vi "KB-C Chart.vi"(9 "P Chart Select":string(combo)="ITEM31(Offset)O-I", 10 "ALL Tolerance Param":string[][](table)=[["Null", "Null", "Null", "Null", "Null", "Null", "Null", "Null", "Null"], ["Null", "Null", "Null", "Null", "Null", "Null", "Null", "Null", "Null"], ["Null", "Null", "Null", "Null", "Null", "Null", "Null", "Null", "Null"], ["Null", "Null", "Null", "Null", "Null", "Null", "Null", "Null", "Null"], ["Null", "Null", "Null", "Null", "Null", "Null", "Null", "Null", "Null"], ["Null", "Null", "Null", "Null", "Null", "Null", "Null", "Null", "Null"], ["Null", "Null", "Null", "Null", "Null", "Null", "Null", "Null", "Null"], ["Null", "Null", "Null", "Null", "Null", "Null", "Null", "Null", "Null"], ["Null", "Null", "Null", "Null", "Null", "Null", "Null", "Null", "Null"], ["Null", "Null", "Null", "Null", "Null", "Null", "Null", "Null", "Null"], ["Null", "Null", "Null", "Null", "Null", "Null", "Null", "Null", "Null"], ["Null", "Null", "Null", "Null", "Null", "Null", "Null", "Null", "Null"], ["Null", "Null", "Null", "Null", "Null", "Null", "Null", "Null", "Null"], ["Null", "Null", "Null", "Null", "Null", "Null", "Null", "Null", "Null"], ["Null", "Null", "Null", "Null", "Null", "Null", "Null", "Null", "Null"], ["Null", "Null", "Null", "Null", "Null", "Null", "Null", "Null", "Null"], ["Null", "Null", "Null", "Null", "Null", "Null", "Null", "Null", "Null"], ["Null", "Null", "Null", "Null", "Null", "Null", "Null", "Null", "Null"], ["Null", "Null", "Null", "Null", "Null", "Null", "Null", "Null", "Null"], ["Null", "Null", "Null", "Null", "Null", "Null", "Null", "Null", "Null"], ["Null", "Null", "Null", "Null", "Null", "Null", "Null", "Null", "Null"], ["Null", "Null", "Null", "Null", "Null", "Null", "Null", "Null", "Null"], ["Null", "Null", "Null", "Null", "Null", "Null", "Null", "Null", "Null"], ["Null", "Null", "Null", "Null", "Null", "Null", "Null", "Null", "Null"], ["Null", "Null", "Null", "Null", "Null", "Null", "Null", "Null", "Null"], ["Null", "Null", "Null", "Null", "Null", "Null", "Null", "Null", "Null"], ["Null", "Null", "Null", "Null", "Null", "Null", "Null", "Null", "Null"], ["Null", "Null", "Null", "Null", "Null", "Null", "Null", "Null", "Null"], ["Null", "Null", "Null", "Null", "Null", "Null", "Null", "Null", "Null"], ["Null", "Null", "Null", "Null", "Null", "Null", "Null", "Null", "Null"], ["Null", "Null", "Null", "Null", "Null", "Null", "Null", "Null", "Null"], ["Null", "Null", "Null", "Null", "Null", "Null", "Null", "Null", "Null"], ["Null", "Null", "Null", "Null", "Null", "Null", "Null", "Null", "Null"]], 11 "Data":string[][](table)=[["Barcode", "StartTime", "Result", "ProductColor", "ITEM1 Result", "ITEM1(Offset)O-I", "ITEM1(Offset)I", "ITEM1(Offset)O", "ITEM1同心度", "ITEM1颜色", "ITEM1是否漏装", "ITEM2 Result", "ITEM2(Offset)O-I", "ITEM2(Offset)I", "ITEM2(Offset)O", "ITEM2同心度", "ITEM2颜色", "ITEM2是否漏装", "ITEM3 Result", "ITEM3(Offset)O-I", "ITEM3(Offset)I", "ITEM3(Offset)O", "ITEM3同心度", "ITEM3颜色", "ITEM3是否漏装", "ITEM4 Result", "ITEM4(Offset)O-I", "ITEM4(Offset)I", "ITEM4(Offset)O", "ITEM4同心度", "ITEM4颜色", "ITEM4是否漏装", "ITEM5 Result", "ITEM5(Offset)O-I", "ITEM5(Offset)I", "ITEM5(Offset)O", "ITEM5同心度", "ITEM5颜色", "ITEM5是否漏装", "ITEM6 Result", "ITEM6(Offset)O-I", "ITEM6(Offset)I", "ITEM6(Offset)O", "ITEM6同心度", "ITEM6颜色", "ITEM6是否漏装", "ITEM7 Result", "ITEM7(Offset)O-I", "ITEM7(Offset)I", "ITEM7(Offset)O", "ITEM7同心度", "ITEM7颜色", "ITEM7是否漏装", "ITEM8 Result", "ITEM8(Offset)O-I", "ITEM8(Offset)I", "ITEM8(Offset)O", "ITEM8同心度", "ITEM8颜色", "ITEM8是否漏装", "ITEM9 Result", "ITEM9(Offset)O-I", "ITEM9(Offset)I", "ITEM9(Offset)O", "ITEM9同心度", "ITEM9颜色", "ITEM9是否漏装", "ITEM10 Result", "ITEM10(Offset)O-I", "ITEM10(Offset)I", "ITEM10(Offset)O", "ITEM10同心度", "ITEM10颜色", "ITEM10是否漏装", "ITEM11 Result", "ITEM11(Offset)O-I", "ITEM11(Offset)I", "ITEM11(Offset)O", "ITEM11同心度", "ITEM11颜色", "ITEM11是否漏装", "ITEM12 Result", "ITEM12(Offset)O-I", "ITEM12(Offset)I", "ITEM12(Offset)O", "ITEM12同心度", "ITEM12颜色", "ITEM12是否漏装", "ITEM13 Result", "ITEM13(Offset)O-I", "ITEM13(Offset)I", "ITEM13(Offset)O", "ITEM13同心度", "ITEM13颜色", "ITEM13是否漏装", "ITEM14 Result", "ITEM14(Offset)O-I", "ITEM14(Offset)I", "ITEM14(Offset)O", "ITEM14同心度", "ITEM14颜色", "ITEM14是否漏装", "ITEM15 Result", "ITEM15(Offset)O-I", "ITEM15(Offset)I", "ITEM15(Offset)O", "ITEM15同心度", "ITEM15颜色", "ITEM15是否漏装", "ITEM16 Result", "ITEM16(Offset)O-I", "ITEM16(Offset)I", "ITEM16(Offset)O", "ITEM16同心度", "ITEM16颜色", "ITEM16是否漏装", "ITEM17 Result", "ITEM17(Offset)O-I", "ITEM17(Offset)I", "ITEM17(Offset)O", "ITEM17同心度", "ITEM17颜色", "ITEM17是否漏装", "ITEM18 Result", "ITEM18(Offset)O-I", "ITEM18(Offset)I", "ITEM18(Offset)O", "ITEM18同心度", "ITEM18颜色", "ITEM18是否漏装", "ITEM19 Result", "ITEM19(Offset)O-I", "ITEM19(Offset)I", "ITEM19(Offset)O", "ITEM19同心度", "ITEM19颜色", "ITEM19是否漏装", "ITEM20 Result", "ITEM20(Offset)O-I", "ITEM20(Offset)I", "ITEM20(Offset)O", "ITEM20同心度", "ITEM20颜色", "ITEM20是否漏装", "ITEM21 Result", "ITEM21(Offset)O-I", "ITEM21(Offset)I", "ITEM21(Offset)O", "ITEM21同心度", "ITEM21颜色", "ITEM21是否漏装", "ITEM22 Result", "ITEM22(Offset)O-I", "ITEM22(Offset)I", "ITEM22(Offset)O", "ITEM22同心度", "ITEM22颜色", "ITEM22是否漏装", "ITEM23 Result", "ITEM23(Offset)O-I", "ITEM23(Offset)I", "ITEM23(Offset)O", "ITEM23同心度", "ITEM23颜色", "ITEM23是否漏装", "ITEM24 Result", "ITEM24(Offset)O-I", "ITEM24(Offset)I", "ITEM24(Offset)O", "ITEM24同心度", "ITEM24颜色", "ITEM24是否漏装", "ITEM25 Result", "ITEM25(Offset)O-I", "ITEM25(Offset)I", "ITEM25(Offset)O", "ITEM25同心度", "ITEM25颜色", "ITEM25是否漏装", "ITEM26 Result", "ITEM26(Offset)O-I", "ITEM26(Offset)I", "ITEM26(Offset)O", "ITEM26同心度", "ITEM26颜色", "ITEM26是否漏装", "ITEM27 Result", "ITEM27(Offset)O-I", "ITEM27(Offset)I", "ITEM27(Offset)O", "ITEM27同心度", "ITEM27颜色", "ITEM27是否漏装", "ITEM28 Result", "ITEM28(Offset)O-I", "ITEM28(Offset)I", "ITEM28(Offset)O", "ITEM28同心度", "ITEM28颜色", "ITEM28是否漏装", "ITEM29 Result", "ITEM29(Offset)O-I", "ITEM29(Offset)I", "ITEM29(Offset)O", "ITEM29同心度", "ITEM29颜色", "ITEM29是否漏装", "ITEM30 Result", "ITEM30(Offset)O-I", "ITEM30(Offset)I", "ITEM30(Offset)O", "ITEM30同心度", "ITEM30颜色", "ITEM30是否漏装", "ITEM31 Result", "ITEM31(Offset)O-I", "ITEM31(Offset)I", "ITEM31(Offset)O", "ITEM31同心度", "ITEM31颜色", "ITEM31是否漏装"], ["3434", "2016-09-24 08:24:53 +0800", "NG", "白色", "OK", "0.040", "0.013", "Null", "0.061", "金色", "无漏装", "OK", "0.059", "0.016", "Null", "0.031", "金色", "无漏装", "OK", "0.042", "0.002", "Null", "0.031", "金色", "无漏装", "OK", "0.056", "0.016", "Null", "0.019", "金色", "无漏装", "OK", "0.037", "0.017", "Null", "0.024", "金色", "无漏装", "OK", "0.059", "0.019", "Null", "0.028", "金色", "无漏装", "OK", "Null", "Null", "Null", "0", "银色", "无漏装", "OK", "Null", "Null", "Null", "0", "银色", "无漏装", "OK", "Null", "Null", "Null", "0", "银色", "无漏装", "OK", "Null", "Null", "Null", "0", "银色", "无漏装", "OK", "0.106", "0.000", "Null", "0.039", "金色", "无漏装", "OK", "0.099", "0.012", "Null", "0.060", "金色", "无漏装", "OK", "0.071", "0.006", "Null", "0.064", "金色", "无漏装", "OK", "0.086", "0.020", "Null", "0.027", "金色", "无漏装", "OK", "0.098", "0.005", "Null", "0.047", "金色", "无漏装", "高度差NG", "-0.027", "0.000", "Null", "0.067", "金色", "无漏装", "OK", "0.081", "0.002", "Null", "0.050", "金色", "无漏装", "OK", "0.102", "0.016", "Null", "0.018", "金色", "无漏装", "OK", "0.154", "0.013", "Null", "0.048", "金色", "无漏装", "OK", "0.040", "0.004", "Null", "0.036", "金色", "无漏装", "OK", "0.065", "0.014", "Null", "0.030", "金色", "无漏装", "OK", "0.205", "0.004", "1.260", "0.015", "金色", "无漏装", "高度差NG", "0.302", "0.006", "0.921", "0.023", "金色", "无漏装", "OK", "0.150", "0.009", "1.375", "0.018", "金色", "无漏装", "高度差NG", "0.267", "0.006", "0.913", "0.034", "金色", "无漏装", "OK", "0.147", "0.016", "0.936", "0.048", "金色", "无漏装", "OK", "0.198", "0.012", "1.345", "0.003", "金色", "无漏装", "高度差NG", "0.350", "0.017", "1.198", "0.037", "金色", "无漏装", "高度差NG", "0.387", "0.011", "0.924", "0.015", "金色", "无漏装", "OK", "0.125", "0.007", "0.962", "0.023", "金色", "无漏装", "高度差NG", "0.289", "0.014", "1.281", "0.021", "金色", "无漏装"]]) -> (3 "结果直方图":dbl[][](graph)=[[0.0, 0.136, 0.145, 0.129, 0.138, 0.133, 0.115, 0.126, 0.122, 0.132, 0.133, 0.133, 0.113, 0.108, 0.111, 0.181, 0.185, 0.182, 0.224, 0.217, 0.221, 0.187, 0.192, 0.188, 0.187, 0.188, 0.19, 0.137, 0.136, 0.134, 0.202, 0.202, 0.206, 0.037, 0.038, 0.036], [0.25, 0.25, 0.25, 0.25, 0.25, 0.25, 0.25, 0.25, 0.25, 0.25, 0.25, 0.25, 0.25, 0.25, 0.25, 0.25, 0.25, 0.25, 0.25, 0.25, 0.25, 0.25, 0.25, 0.25, 0.25, 0.25, 0.25, 0.25, 0.25, 0.25, 0.25, 0.25, 0.25, 0.25, 0.25, 0.25], [0.0, 0.0, 0.0, 0.0, 0.0, 0.0, 0.0, 0.0, 0.0, 0.0, 0.0, 0.0, 0.0, 0.0, 0.0, 0.0, 0.0, 0.0, 0.0, 0.0, 0.0, 0.0, 0.0, 0.0, 0.0, 0.0, 0.0, 0.0, 0.0, 0.0, 0.0, 0.0, 0.0, 0.0, 0.0, 0.0], [0.125, 0.125, 0.125, 0.125, 0.125, 0.125, 0.125, 0.125, 0.125, 0.125, 0.125, 0.125, 0.125, 0.125, 0.125, 0.125, 0.125, 0.125, 0.125, 0.125, 0.125, 0.125, 0.125, 0.125, 0.125, 0.125, 0.125, 0.125, 0.125, 0.125, 0.125, 0.125, 0.125, 0.125, 0.125, 0.125]])   [LabVIEW 2015]
panel:
  out "添加的数组 2":i32[](array[numeric])
  out "数字":dbl[](array[numeric])
  out "添加的数组":i32[](array[numeric])
  out "大小 2":i32
  out "大小":i32
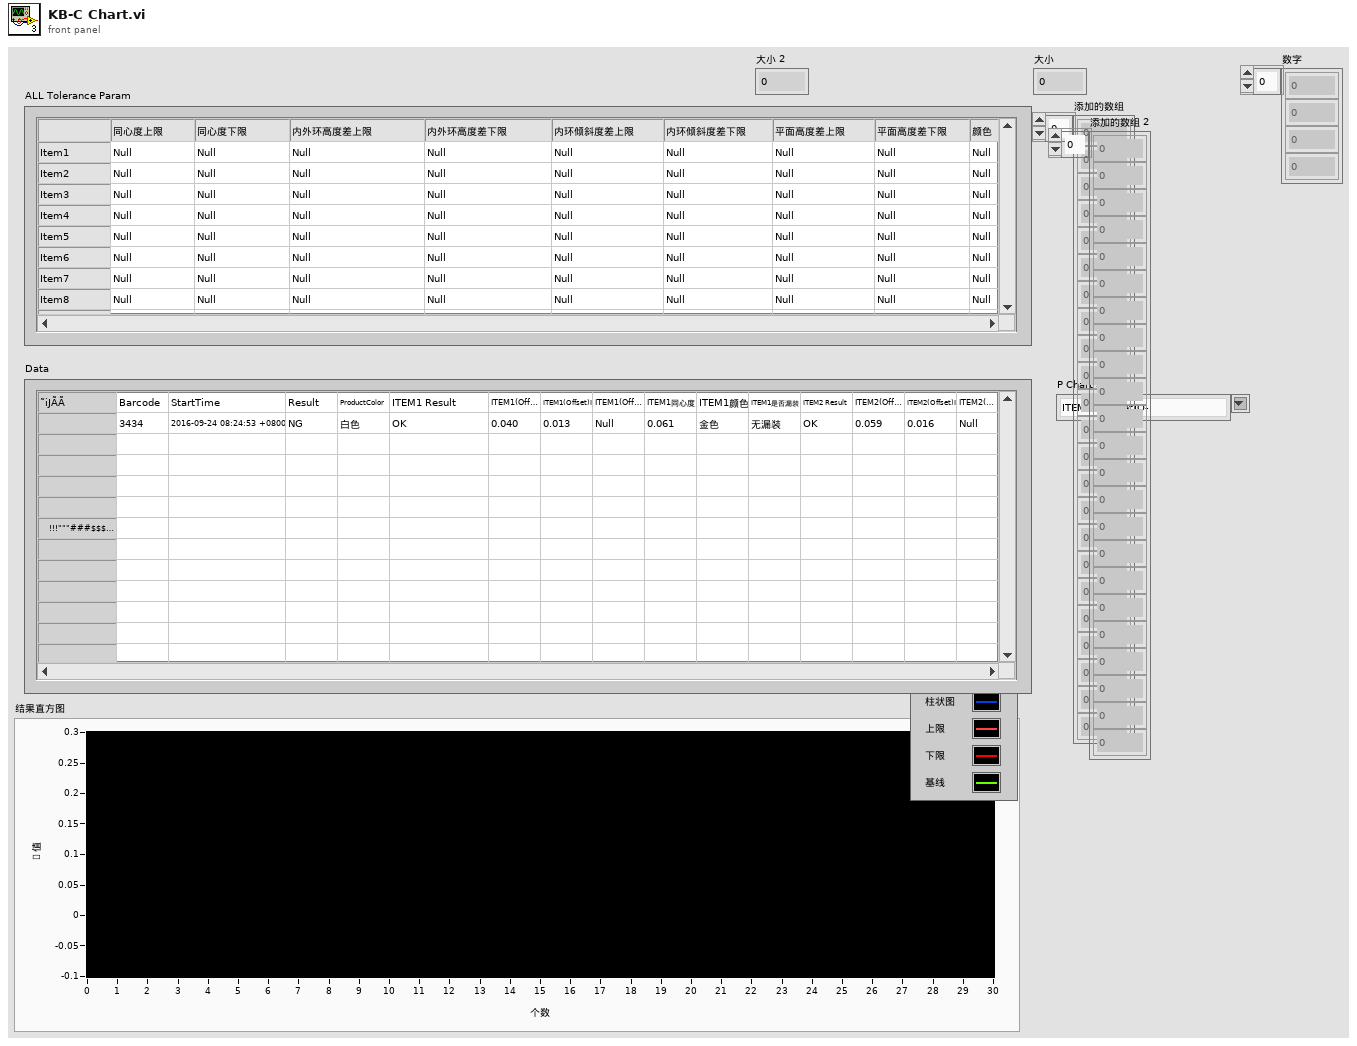
[diagram p1: front panel]
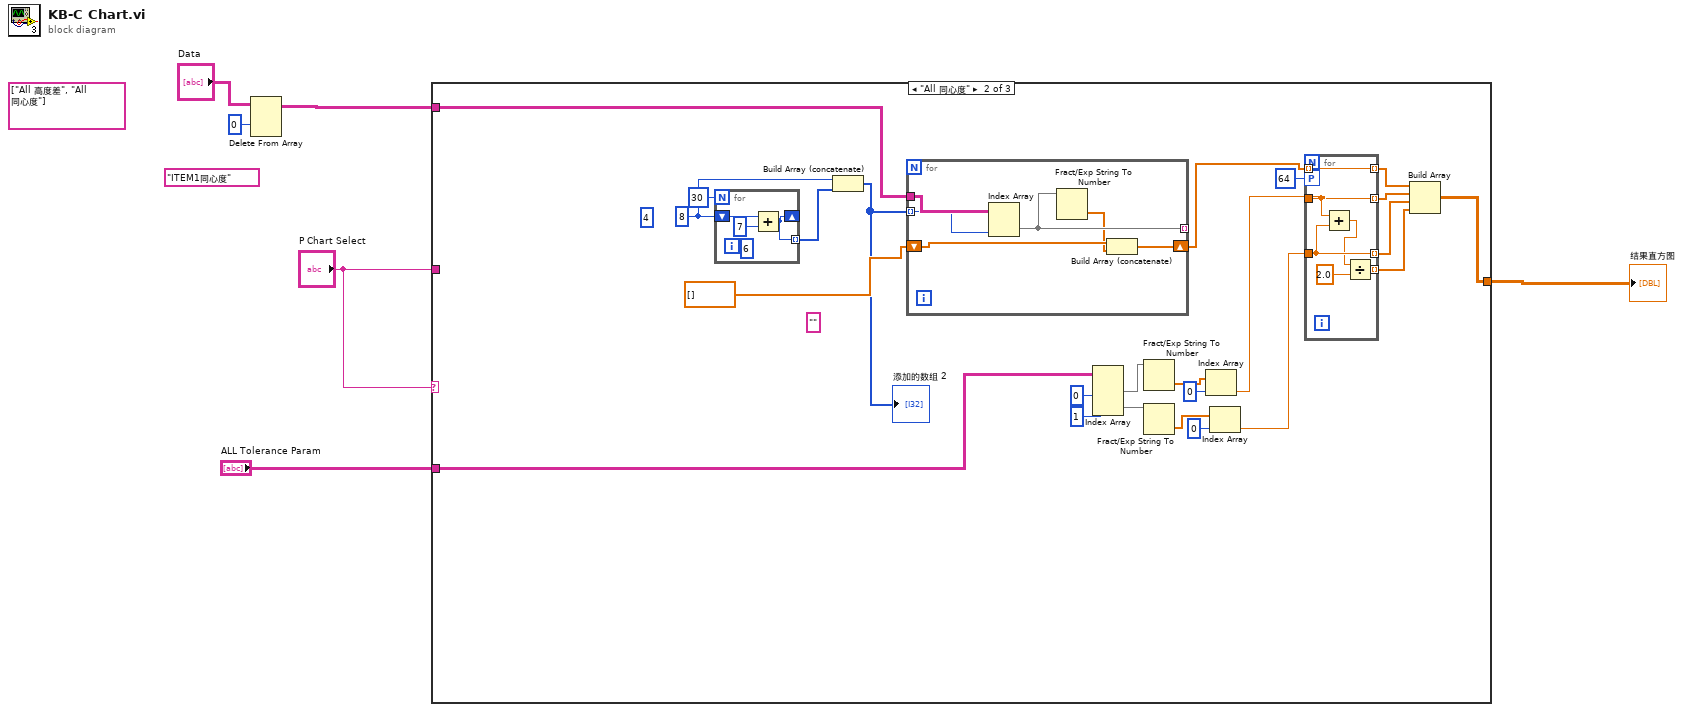
[diagram p0: block diagram]
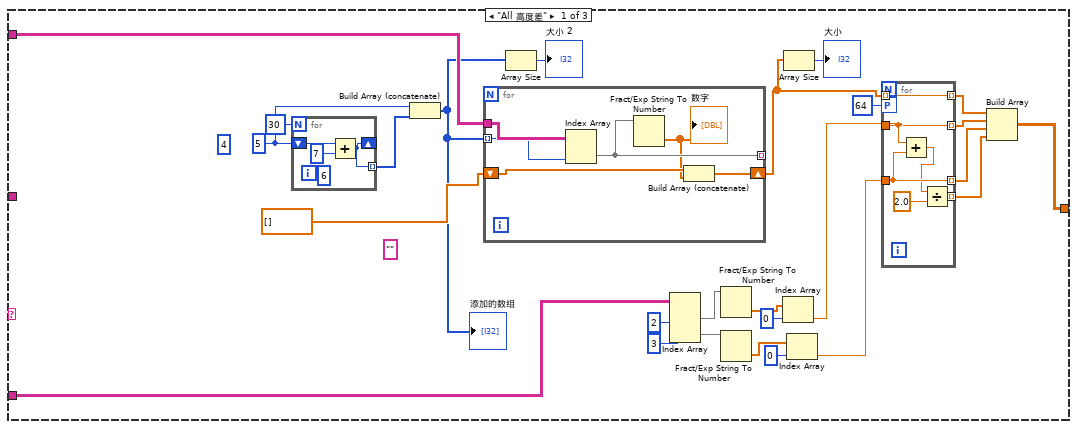
[diagram p2: hidden frame]
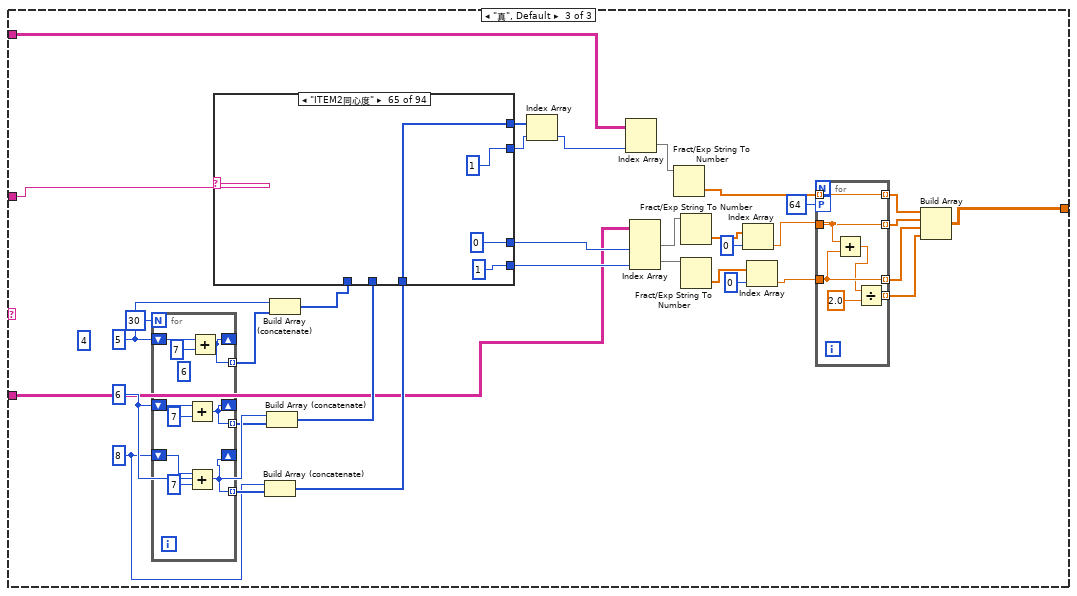
[diagram p3: hidden frame]
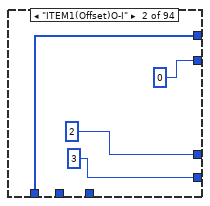
[diagram p5: hidden frame]
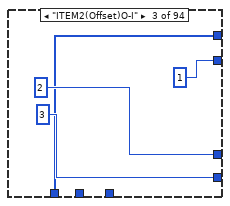
[diagram p6: hidden frame]
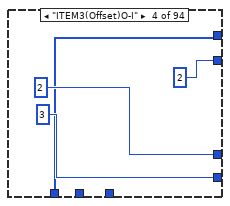
[diagram p7: hidden frame]
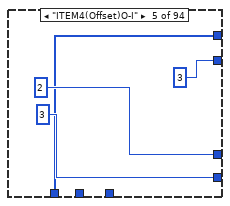
[diagram p8: hidden frame]
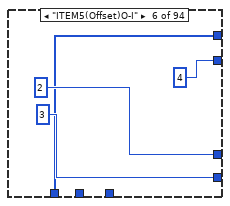
[diagram p9: hidden frame]
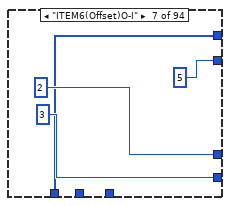
[diagram p10: hidden frame]
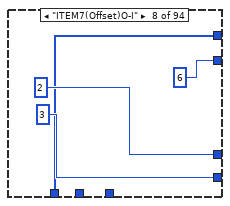
[diagram p11: hidden frame]
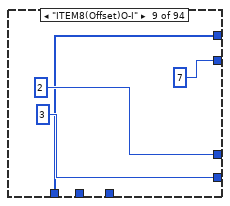
[diagram p12: hidden frame]
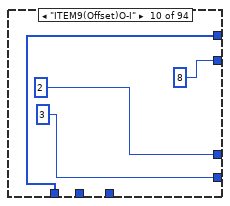
[diagram p13: hidden frame]
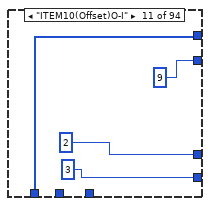
[diagram p14: hidden frame]
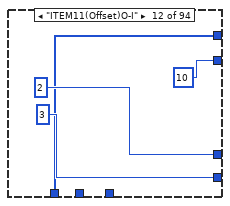
[diagram p15: hidden frame]
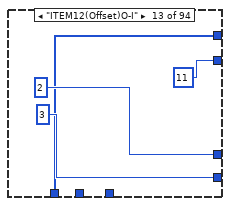
[diagram p16: hidden frame]
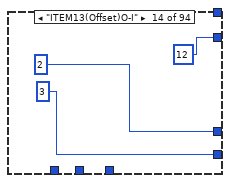
[diagram p17: hidden frame]
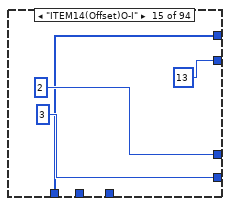
[diagram p18: hidden frame]
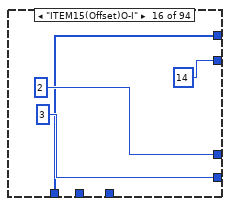
[diagram p19: hidden frame]
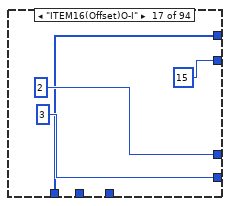
[diagram p20: hidden frame]
diagram:
  (unwired) string[] ["All 高度差", "All 同心度"] ("元素")
  (unwired) "ITEM1同心度" ("P Chart Select 2")
  n1 = Delete From Array(array="Data", index (row)=0 ("索引 (行)")) -> (array with subset deleted=w1:string[][])  [unwired: 2 in, 1 out]
  n2 = case shown="\"All 同心度\"" "P Chart Select" {
    tunnel: [w11 w50 w107] -> w6
    tunnel: w1 -> [w29 w68 w95]
    tunnel: "P Chart Select" -> [_ _ w94]
    tunnel: "ALL Tolerance Param" -> [w22 w61 w87]
    frame "All 高度差" {
      (unwired) ""
      (unwired) 4
      w30 = 5
      n3 = for {
        N: 30 -> [_]
        shift-right: [w45] -> _
        shift-left: w30 -> [w47]
        tunnel: [w45] -> w31 mode=indexing
        (unwired) 6 ("y")
        n4 = Add(x=w47, y=7) -> (x+y=w45:i32)
      }
      n5 = Build Array (concatenate)(w30, w31) -> (w7:i32[])
      "添加的数组" <- w7
      n6 = for {
        tunnel: w7 -> [w43] mode=indexing
        tunnel: w29 -> [w44]
        tunnel: [w41] -> _ mode=indexing
        shift-right: [w39] -> w10
        shift-left: dbl[] [] -> [w42]
        n7 = Index Array(array=w44, index (col)=w43) -> (element=w41:string[])  [unwired: 1 in]
        n8 = Fract/Exp String To Number ("分数/指数字符串至数值转换")(string=w41) -> (number=w40:dbl[])  [unwired: 3 in, 1 out]
        "数字" <- w40
        n9 = Build Array (concatenate)(w42, w40) -> (w39:dbl[])
      }
      n10 = Array Size(array=w7) -> (size(s)=→"大小 2":i32)
      n11 = Index Array(array=w22, index (col) #1=2 ("禁用的索引 (列)"), index (col) #2=3 ("索引 (列)")) -> (element #1=w28:string[], element #2=w27:string[])  [unwired: 2 in]
      n12 = Fract/Exp String To Number(string=w28) -> (number=w26:dbl[])  [unwired: 3 in, 1 out]
      n13 = Fract/Exp String To Number(string=w27) -> (number=w25:dbl[])  [unwired: 3 in, 1 out]
      n14 = Index Array(array=w26, index=0 ("索引")) -> (element=w13:dbl)
      n15 = Array Size(array=w10) -> (size(s)=→"大小":i32)
      n16 = Index Array(array=w25, index=0 ("索引")) -> (element=w12:dbl)
      n17 = for {
        tunnel: w10 -> [w38] mode=indexing
        tunnel: w13 -> [w37]
        tunnel: w12 -> [w36]
        tunnel: [w38] -> w18 mode=indexing
        tunnel: [w37] -> w17 mode=indexing
        tunnel: [w36] -> w16 mode=indexing
        tunnel: [w33] -> w15 mode=indexing
        workers-P: 64 -> [_]
        n18 = Add(x=w37, y=w36) -> (x+y=w35:dbl)
        n19 = Divide(x=w35, y=2.0) -> (x/y=w33:dbl)
      }
      n20 = Build Array(w18, w17, w16, w15) -> (w11:dbl[][])
    }
    frame "All 同心度" {
      (unwired) ""
      (unwired) 4
      w69 = 8
      n21 = for {
        N: 30 -> [_]
        shift-right: [w84] -> _
        shift-left: w69 -> [w86]
        tunnel: [w84] -> w70 mode=indexing
        (unwired) 6 ("y")
        n22 = Add(x=w86, y=7) -> (x+y=w84:i32)
      }
      n23 = Build Array (concatenate)(w69, w70) -> (w48:i32[])
      "添加的数组 2" <- w48
      n24 = for {
        tunnel: w48 -> [w82] mode=indexing
        tunnel: w68 -> [w83]
        tunnel: [w80] -> _ mode=indexing
        shift-right: [w78] -> w49
        shift-left: dbl[] [] -> [w81]
        n25 = Index Array(array=w83, index (col)=w82) -> (element=w80:string[])  [unwired: 1 in]
        n26 = Fract/Exp String To Number ("分数/指数字符串至数值转换")(string=w80) -> (number=w79:dbl[])  [unwired: 3 in, 1 out]
        n27 = Build Array (concatenate)(w81, w79) -> (w78:dbl[])
      }
      n28 = Index Array(array=w61, index (col) #1=0 ("禁用的索引 (列)"), index (col) #2=1 ("索引 (列)")) -> (element #1=w67:string[], element #2=w66:string[])  [unwired: 2 in]
      n29 = Fract/Exp String To Number(string=w67) -> (number=w65:dbl[])  [unwired: 3 in, 1 out]
      n30 = Fract/Exp String To Number(string=w66) -> (number=w64:dbl[])  [unwired: 3 in, 1 out]
      n31 = Index Array(array=w65, index=0 ("索引")) -> (element=w52:dbl)
      n32 = Index Array(array=w64, index=0 ("索引")) -> (element=w51:dbl)
      n33 = for {
        tunnel: w49 -> [w77] mode=indexing
        tunnel: w52 -> [w76]
        tunnel: w51 -> [w75]
        tunnel: [w77] -> w57 mode=indexing
        tunnel: [w76] -> w56 mode=indexing
        tunnel: [w75] -> w55 mode=indexing
        tunnel: [w72] -> w54 mode=indexing
        workers-P: 64 -> [_]
        n34 = Add(x=w76, y=w75) -> (x+y=w74:dbl)
        n35 = Divide(x=w74, y=2.0) -> (x/y=w72:dbl)
      }
      n36 = Build Array(w57, w56, w55, w54) -> (w50:dbl[][])
    }
    frame "真", Default {
      (unwired) 4
      w89 = 8
      w93 = 6
      w100 = 5
      n37 = for {
        N: 30 -> [_]
        shift-right: [w127] -> _
        shift-left: w100 -> [w129]
        tunnel: [w127] -> w101 mode=indexing
        shift-right: [w124] -> _
        shift-left: w93 -> [w125]
        tunnel: [w124] -> w92 mode=indexing
        shift-right: [w121] -> _
        shift-left: w89 -> [w122]
        tunnel: [w121] -> w90 mode=indexing
        (unwired) 6 ("y")
        n38 = Add(x=w125, y=7) -> (x+y=w124:i32)
        n39 = Add(x=w122, y=7) -> (x+y=w121:i32)
        n40 = Add(x=w129, y=7) -> (x+y=w127:i32)
      }
      n41 = Build Array (concatenate)(w89, w90) -> (w88:i32[])
      n42 = Build Array (concatenate)(w93, w92) -> (w91:i32[])
      n43 = Build Array (concatenate)(w100, w101) -> (w97:i32[])
      n44 = case shown="\"ITEM2同心度\"" w94 {
        tunnel: [_ 0 1 2 3 4 5 6 7 8 9 10 11 12 13 14 15 16 17 18 19 20 2 22 23 24 25 26 27 28 29 30 0 1 2 3 4 5 6 7 8 9 10 11 12 13 14 15 16 17 18 19 20 21 22 23 24 25 26 27 28 29 30 0 1 2 3 4 5 6 7 8 9 10 11 12 13 14 15 16 17 18 19 20 21 22 23 24 25 26 27 28 29 30] -> w99
        tunnel: [_ 2 2 2 2 2 2 2 2 2 2 2 2 2 2 2 2 2 2 2 2 2 2 2 2 2 2 2 2 2 2 2 4 4 4 4 4 4 4 4 4 4 4 4 4 4 4 4 4 4 4 4 4 4 4 4 4 4 4 4 4 4 4 0 0 0 0 0 0 0 0 0 0 0 0 0 0 0 0 0 0 0 0 0 0 0 0 0 0 0 0 0 0 0] -> w106
        tunnel: [_ 3 3 3 3 3 3 3 3 3 3 3 3 3 3 3 3 3 3 3 3 3 3 3 3 3 3 3 3 3 3 3 5 5 5 5 5 5 5 5 5 5 5 5 5 5 5 5 5 5 5 5 5 5 5 5 5 5 5 5 5 5 5 1 1 1 1 1 1 1 1 1 1 1 1 1 1 1 1 1 1 1 1 1 1 1 1 1 1 1 1 1 1 1] -> w105
        tunnel: w97 -> [_ w136 w140 w144 w148 w152 w156 w160 w164 w168 w172 w176 w180 _ w187 w191 w195 w199 w203 w207 w211 w215 w219 w223 w227 w231 w235 w239 w243 w247 w251 w255 _ _ _ _ _ _ _ _ _ _ _ _ _ _ _ _ _ _ _ _ _ _ _ _ _ _ _ _ _ _ _ _ _ _ _ _ _ _ _ _ _ _ _ _ _ _ _ _ _ _ _ _ _ _ _ _ _ _ _ _ _ _]
        tunnel: [_ w136 w140 w144 w148 w152 w156 w160 w164 w168 w172 w176 w180 _ w187 w191 w195 w199 w203 w207 w211 w215 w219 w223 w227 w231 w235 w239 w243 w247 w251 w255 w259 w263 w267 w271 w275 w279 w283 w287 w291 w295 w299 w303 w307 w311 w315 w319 w323 w327 w331 w335 w339 w343 w347 w351 w355 w359 w363 w367 w371 w375 w379 w383 w387 w391 w395 w399 w403 w407 w411 w415 w419 w423 w427 w431 w435 w439 w443 w447 w451 w455 w459 w463 w467 w471 w475 w479 w483 w487 w491 w495 w499 w503] -> w96
        tunnel: w91 -> [_ _ _ _ _ _ _ _ _ _ _ _ _ _ _ _ _ _ _ _ _ _ _ _ _ _ _ _ _ _ _ _ w259 w263 w267 w271 w275 w279 w283 w287 w291 w295 w299 w303 w307 w311 w315 w319 w323 w327 w331 w335 w339 w343 w347 w351 w355 w359 w363 w367 w371 w375 w379 _ _ _ _ _ _ _ _ _ _ _ _ _ _ _ _ _ _ _ _ _ _ _ _ _ _ _ _ _ _ _]
        tunnel: w88 -> [_ _ _ _ _ _ _ _ _ _ _ _ _ _ _ _ _ _ _ _ _ _ _ _ _ _ _ _ _ _ _ _ _ _ _ _ _ _ _ _ _ _ _ _ _ _ _ _ _ _ _ _ _ _ _ _ _ _ _ _ _ _ _ w383 w387 w391 w395 w399 w403 w407 w411 w415 w419 w423 w427 w431 w435 w439 w443 w447 w451 w455 w459 w463 w467 w471 w475 w479 w483 w487 w491 w495 w499 w503]
        frame "假", Default {
        }
        frame "ITEM1(Offset)O-I" {
        }
        frame "ITEM2(Offset)O-I" {
        }
        frame "ITEM3(Offset)O-I" {
        }
        frame "ITEM4(Offset)O-I" {
        }
        frame "ITEM5(Offset)O-I" {
        }
        frame "ITEM6(Offset)O-I" {
        }
        frame "ITEM7(Offset)O-I" {
        }
        frame "ITEM8(Offset)O-I" {
        }
        frame "ITEM9(Offset)O-I" {
        }
        frame "ITEM10(Offset)O-I" {
        }
        frame "ITEM11(Offset)O-I" {
        }
        frame "ITEM12(Offset)O-I" {
        }
        frame "ITEM13(Offset)O-I" {
        }
        frame "ITEM14(Offset)O-I" {
        }
        frame "ITEM15(Offset)O-I" {
        }
        frame "ITEM16(Offset)O-I" {
        }
        frame "ITEM17(Offset)O-I" {
        }
        frame "ITEM18(Offset)O-I" {
        }
        frame "ITEM19(Offset)O-I" {
        }
        frame "ITEM20(Offset)O-I" {
        }
        frame "ITEM21(Offset)O-I" {
        }
        frame "ITEM22(Offset)O-I" {
        }
        frame "ITEM23(Offset)O-I" {
        }
        frame "ITEM24(Offset)O-I" {
        }
        frame "ITEM25(Offset)O-I" {
        }
        frame "ITEM26(Offset)O-I" {
        }
        frame "ITEM27(Offset)O-I" {
        }
        frame "ITEM28(Offset)O-I" {
        }
        frame "ITEM29(Offset)O-I" {
        }
        frame "ITEM30(Offset)O-I" {
        }
        frame "ITEM31(Offset)O-I" {
        }
        frame "ITEM1(Offset)I" {
        }
        frame "ITEM2(Offset)I" {
        }
        frame "ITEM3(Offset)I" {
        }
        frame "ITEM4(Offset)I" {
        }
        frame "ITEM5(Offset)I" {
        }
        frame "ITEM6(Offset)I" {
        }
        frame "ITEM7(Offset)I" {
        }
        frame "ITEM8(Offset)I" {
        }
        frame "ITEM9(Offset)I" {
        }
        frame "ITEM10(Offset)I" {
        }
        frame "ITEM11(Offset)I" {
        }
        frame "ITEM12(Offset)I" {
        }
        frame "ITEM13(Offset)I" {
        }
        frame "ITEM14(Offset)I" {
        }
        frame "ITEM15(Offset)I" {
        }
        frame "ITEM16(Offset)I" {
        }
        frame "ITEM17(Offset)I" {
        }
        frame "ITEM18(Offset)I" {
        }
        frame "ITEM19(Offset)I" {
        }
        frame "ITEM20(Offset)I" {
        }
        frame "ITEM21(Offset)I" {
        }
        frame "ITEM22(Offset)I" {
        }
        frame "ITEM23(Offset)I" {
        }
        frame "ITEM24(Offset)I" {
        }
        frame "ITEM25(Offset)I" {
        }
        frame "ITEM26(Offset)I" {
        }
        frame "ITEM27(Offset)I" {
        }
        frame "ITEM28(Offset)I" {
        }
        frame "ITEM29(Offset)I" {
        }
        frame "ITEM30(Offset)I" {
        }
        frame "ITEM31(Offset)I" {
        }
        frame "ITEM1同心度" {
        }
        frame "ITEM2同心度" {
        }
        frame "ITEM3同心度" {
        }
        frame "ITEM4同心度" {
        }
        frame "ITEM5同心度" {
        }
        frame "ITEM6同心度" {
        }
        frame "ITEM7同心度" {
        }
        frame "ITEM8同心度" {
        }
        frame "ITEM9同心度" {
        }
        frame "ITEM10同心度" {
        }
        frame "ITEM11同心度" {
        }
        frame "ITEM12同心度" {
        }
        frame "ITEM13同心度" {
        }
        frame "ITEM14同心度" {
        }
        frame "ITEM15同心度" {
        }
        frame "ITEM16同心度" {
        }
        frame "ITEM17同心度" {
        }
        frame "ITEM18同心度" {
        }
        frame "ITEM19同心度" {
        }
        frame "ITEM20同心度" {
        }
        frame "ITEM21同心度" {
        }
        frame "ITEM22同心度" {
        }
        frame "ITEM23同心度" {
        }
        frame "ITEM24同心度" {
        }
        frame "ITEM25同心度" {
        }
        frame "ITEM26同心度" {
        }
        frame "ITEM27同心度" {
        }
        frame "ITEM28同心度" {
        }
        frame "ITEM29同心度" {
        }
        frame "ITEM30同心度" {
        }
        frame "ITEM31同心度" {
        }
      }
      n45 = Index Array(array=w96, index=w99) -> (element=w98:i32)
      n46 = Index Array(array=w95, index (col)=w98) -> (element=w120:string[])  [unwired: 1 in]
      n47 = Index Array(array=w87, index (col) #1=w106, index (col) #2=w105) -> (element #1=w118:string[], element #2=w117:string[])  [unwired: 2 in]
      n48 = Fract/Exp String To Number(string=w120) -> (number=w119:dbl[])  [unwired: 3 in, 1 out]
      n49 = Fract/Exp String To Number(string=w118) -> (number=w116:dbl[])  [unwired: 3 in, 1 out]
      n50 = Fract/Exp String To Number(string=w117) -> (number=w115:dbl[])  [unwired: 3 in, 1 out]
      n51 = Index Array(array=w116, index=0 ("索引")) -> (element=w112:dbl)
      n52 = Index Array(array=w115, index=0 ("索引")) -> (element=w111:dbl)
      n53 = for {
        tunnel: w119 -> [w135] mode=indexing
        tunnel: w112 -> [w134]
        tunnel: w111 -> [w133]
        tunnel: [w135] -> w110 mode=indexing
        tunnel: [w134] -> w109 mode=indexing
        tunnel: [w133] -> w108 mode=indexing
        tunnel: [w130] -> w104 mode=indexing
        workers-P: 64 -> [_]
        n54 = Add(x=w134, y=w133) -> (x+y=w132:dbl)
        n55 = Divide(x=w132, y=2.0) -> (x/y=w130:dbl)
      }
      n56 = Build Array(w110, w109, w108, w104) -> (w107:dbl[][])
    }
  }
  "结果直方图" <- w6
